vi "get channels.vi"(11 "io configuration in":refnum<class "io configuration.lvclass">) -> (2 "channels":refnum<class "TBM channel.lvclass">[](array[class]), 3 "io configuration out":refnum<class "io configuration.lvclass">)   [LabVIEW 2015, in "io configuration.lvclass"]
uses:
  io configuration.lvclass
  <vilib>/NI/Tag Bus Module Framework/channel/TBM channel.lvclass
  io configuration.lvclass/io configuration.ctl
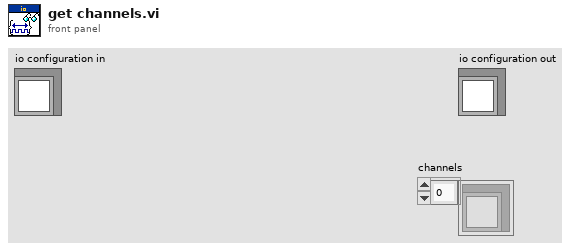
[diagram p1: front panel]
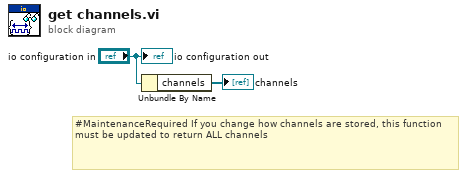
[diagram p0: block diagram]
diagram:
  # "#MaintenanceRequired If you change how channels are stored, this function must be updated to return ALL channels"
  n1 = Unbundle By Name("io configuration in") -> ("channels"=→"channels":refnum<class "TBM channel.lvclass">[])
  "io configuration out" <- "io configuration in"
